vi "LM_Model_Gaussian_MODCA2.vi"(3 "output control":T1, 4 "data":variant, 5 "X":dbl[](array[numeric]), 6 "a":dbl[](array[numeric])) -> (0 "error out":errorcluster, 1 "f'(X,a)":dbl[][](array[numeric]), 2 "f(X,a)":dbl[](array[numeric]))   [LabVIEW 2015]
doc: "This template is the starting point for creating a model function to be passed to the Nonlinear Curve Fit.vi."
uses:
  <vilib>/gmath/NumericalOptimization/LM_output select.ctl
  <vilib>/gmath/NI_Gmath.lvlib
panel:
  # "Corrections in green, see diagram\nhttps://forums.ni.com/t5/LabVIEW/Problem-in-fitting-when-I-am-giving-f-X-a-Partial-derivatives-in/m-p/3301846#M966025"
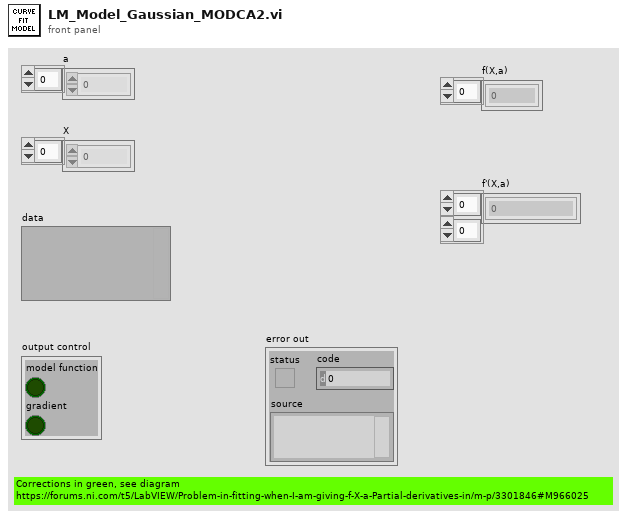
[diagram p1: front panel]
types:
  T1 = typedef "NI_Gmath.lvlib/LM_output select.ctl" = cluster{"model function":bool, "gradient":bool}
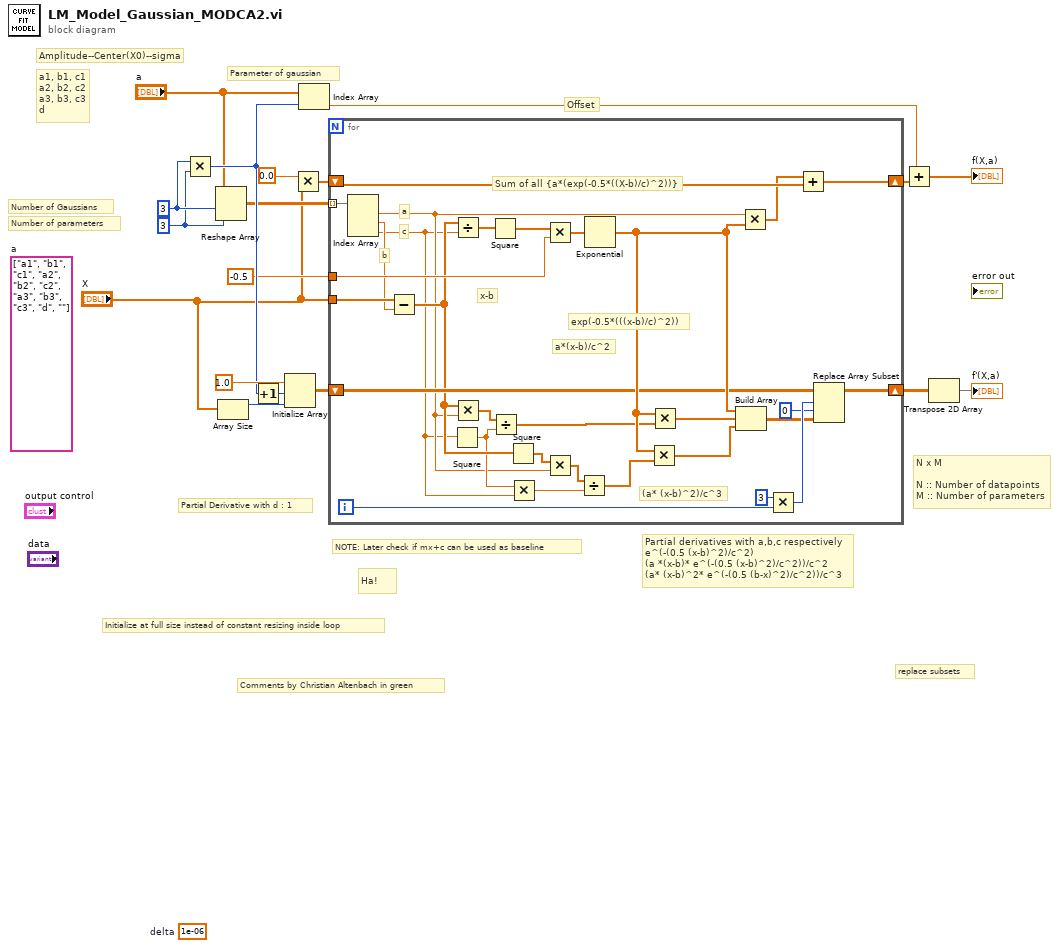
[diagram p0: block diagram]
diagram:
  (unwired) 1e-06  # delta
  (unwired) string[] ["a1", "b1", "c1", "a2", "b2", "c2", "a3", "b3", "c3", "d", ""]  # a
  w17 = 3 ("dimension size")
  w18 = 3 ("dimension size")
  # "Comments by Christian Altenbach in green"
  # "replace subsets"
  # "Initialize at full size instead of constant resizing inside loop"
  # "Ha!"
  # "N x M \n\nN :: Number of datapoints\nM :: Number of parameters"
  # "Partial Derivative with d : 1"
  # "Partial derivatives with a,b,c respectively\ne^(-(0.5 (x-b)^2)/c^2)\n(a *(x-b)* e^(-(0.5 (x-b)^2)/c^2))/c^2\n(a* (x-b)^2* e^(-(0.5 (b-x)^2)/c^2))/c^3"
  # "NOTE: Later check if mx+c can be used as baseline"
  # "Offset"
  # "Amplitude--Center(X0)--sigma"
  # "Parameter of gaussian"
  # "Number of parameters"
  # "Number of Gaussians"
  # "a1, b1, c1\na2, b2, c2\na3, b3, c3\nd"
  n1 = Multiply(x=w18, y=w17) -> (x*y=w11:i32)
  n2 = Reshape Array("a", w18, w17) -> (w7:dbl[][])
  n3 = Array Size(array="X") -> (size(s)=w13:i32)
  n4 = Increment(x=w11) -> (x+1=w10:i32)
  n5 = Initialize Array(1.0 ("element"), w10, w13) -> (w14:dbl[][])
  n6 = Multiply(x=0.0 ("element"), y="X") -> (x*y=w8:dbl[])
  n7 = Index Array(array="a", index=w11) -> (element=w12:dbl)
  n8 = for {
    tunnel: w7 -> [w48] mode=indexing
    tunnel: "X" -> [w47]
    tunnel: -0.5 -> [w46]
    shift-right: [w45] -> w16
    shift-left: w8 -> [w44]
    shift-right: [w33] -> w1
    shift-left: w14 -> [w34]
    i -> [w32]
    # "(a* (x-b)^2)/c^3"
    # "a*(x-b)/c^2"
    # "exp(-0.5*(((x-b)/c)^2))"
    # "x-b"
    # "a"
    # "c"
    # "b"
    # "Sum of all {a*(exp(-0.5*((X-b)/c)^2))}"
    n9 = Index Array(array=w48) -> (element #1=w24:dbl, element #2=w42:dbl, element #3=w23:dbl)  [unwired: 3 in]
    n10 = Subtract(x=w47, y=w42) -> (x-y=w27:dbl[])
    n11 = Square(x=w23) -> (x^2=w25:dbl)
    n12 = Divide ("(x-b1)/c")(x=w27, y=w23) -> (x/y=w41:dbl[])
    n13 = Multiply(x=w27, y=w24) -> (x*y=w39:dbl[])
    n14 = Square(x=w41) -> (x^2=w38:dbl[])
    n15 = Divide(x=w39, y=w25) -> (x/y=w29:dbl[])
    n16 = Square(x=w27) -> (x^2=w26:dbl[])
    n17 = Multiply(x=w25, y=w23) -> (x*y=w22:dbl)
    n18 = Multiply(x=w38, y=w46) -> (x*y=w40:dbl[])
    n19 = Multiply(x=w26, y=w24) -> (x*y=w37:dbl[])
    n20 = Divide(x=w37, y=w22) -> (x/y=w36:dbl[])
    n21 = Exponential(1:w40) -> (0:w35:dbl[])
    n22 = Multiply(x=w35, y=w36) -> (x*y=w28:dbl[])
    n23 = Multiply(x=w35, y=w29) -> (x*y=w19:dbl[])
    n24 = Build Array(w35, w19, w28) -> (w21:dbl[][])
    n25 = Multiply(x=w24, y=w35) -> (x*y=w43:dbl[])
    n26 = Multiply(x=3, y=w32) -> (x*y=w30:i32)
    n27 = Add(x=w43, y=w44) -> (x+y=w45:dbl[])
    n28 = Replace Array Subset(array=w34, new element=w21, index (row)=w30, index (col)=0 ("disabled index (col)")) -> (w33:dbl[][])
  }
  n29 = Add(x=w12, y=w16) -> (x+y=→"f(X,a)":dbl[])
  n30 = Transpose 2D Array(2D array=w1) -> (transposed array=→"f'(X,a)":dbl[][])
